vi "NagleDemo-MessageSender.vi"() -> ()   [LabVIEW 2014]
panel:
  in  "TCP_NODELAY":bool=TRUE caption="false: Nagle alg. ENABLED\ntrue: Nagle alg. DISABLED"
  in  "n iterations":i32=100
  in  "IP address of MessageReflector":string
  out "value":i32
  in  "remote port":u16=5678
  out "error out":errorcluster
  out "roundtrip time (ms)":u32(graph)
  # "This VI demonstrates the effect of having the TCP Nagle algorithm enabled or disabled on  a socket for a particular kind of query/response protocol.\n\nTo run this demo, first run its partner in crime, NagleDemo-MessageSender.vi, on another machine, then run this VI after filling in the IP address of the other machine. Between runs of this VI, toggle the TCP_NODELAY boolean to see the difference."
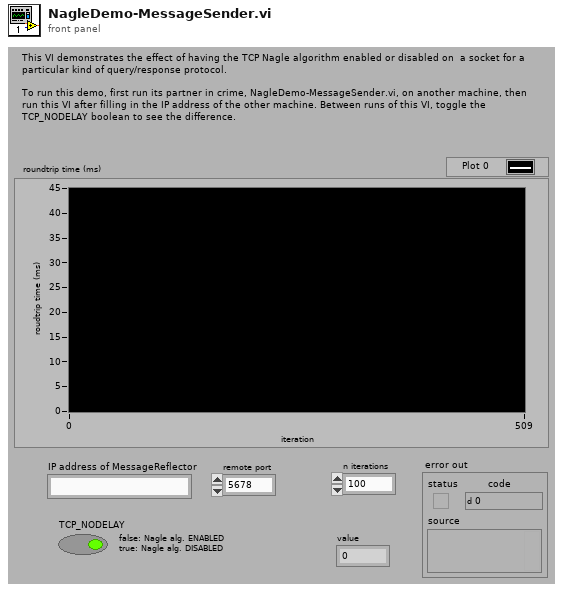
[diagram p1: front panel]
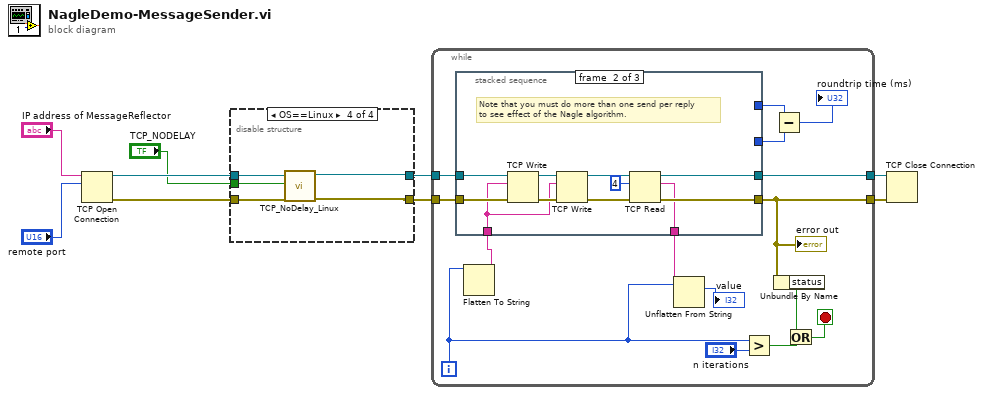
[diagram p0: block diagram]
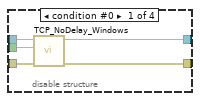
[diagram p2: hidden frame]
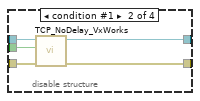
[diagram p3: hidden frame]
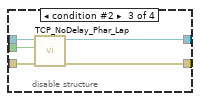
[diagram p4: hidden frame]
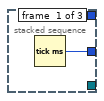
[diagram p5: hidden frame]
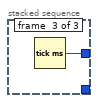
[diagram p6: hidden frame]
diagram:
  n1 = TCP Open Connection(address="IP address of MessageReflector", remote port or service name="remote port") -> (connection ID=w3:refnum<k5>, error out=w1:errorcluster)  [unwired: 3 in]
  n2 = disable-structure shown="OS==Linux" {
    disable-tunnel: [w14 w18 w23 w25] -> w5
    disable-tunnel: [w13 w17 w22 w26] -> w4
    disable-tunnel: w3 -> [w12 w16 w21 w28]
    disable-tunnel: "TCP_NODELAY" -> [w11 w15 w20 w27]
    disable-tunnel: w1 -> [w10 w19 w24 w29]
    frame condition #0 {
      n3 = call "TCP_NoDelay_Windows.vi"("error in (no error)"=w10, "TCP_NODELAY (true)"=w11, "connID"=w12) -> ("error out"=w14:errorcluster, "connID 2"=w13:refnum<k5>)  [unwired: 3 in]
    }
    frame condition #1 {
      n4 = call "TCP_NoDelay_VxWorks.vi"("error in (no error)"=w19, "TCP_NODELAY (true)"=w15, "connID"=w16) -> ("error out"=w18:errorcluster, "connID 2"=w17:refnum<k5>)  [unwired: 3 in]
    }
    frame condition #2 {
      n5 = call "TCP_NoDelay_Phar_Lap.vi"("error in (no error)"=w24, "TCP_NODELAY (true)"=w20, "connID"=w21) -> ("error out"=w23:errorcluster, "connID 2"=w22:refnum<k5>)  [unwired: 3 in]
    }
    frame condition #3 (active) {
      n6 = call "TCP_NoDelay_Linux.vi"("error in (no error)"=w29, "TCP_NODELAY (true)"=w27, "connID"=w28) -> ("error out"=w25:errorcluster, "connID 2"=w26:refnum<k5>)  [unwired: 3 in]
    }
  }
  n7 = while {
    tunnel: w4 -> [w44]
    tunnel: [w43] -> w9
    tunnel: [w39] -> w8
    tunnel: w5 -> [w42]
    i -> [w32]
    stop <- w35 stop-if-true
    n8 = Flatten To String(anything=w32) -> (data string=w34:string)  [unwired: 3 in, 2 out]
    n9 = stacked-sequence {
      tunnel: w44 -> [_ w56 _]
      tunnel: [_ w55 _] -> w43
      tunnel: w42 -> [_ w54 _]
      tunnel: [_ w52 _] -> w39
      tunnel: [w45 _ _] -> w40
      tunnel: [_ _ w57] -> w41
      tunnel: w34 -> [_ w46 _]
      tunnel: [_ w51 _] -> w33
      frame #0 {
        n10 = Tick Count (ms)() -> (millisecond timer value=w45:u32)
      }
      frame #1 {
        # "Note that you must do more than one send per reply\nto see effect of the Nagle algorithm."
        n11 = TCP Write(connection ID=w56, data in=w46, error in (no error)=w54) -> (connection ID out=w50:refnum<k5>, error out=w49:errorcluster)  [unwired: 1 in, 1 out]
        n12 = TCP Write(connection ID=w50, data in=w46, error in (no error)=w49) -> (connection ID out=w47:refnum<k5>, error out=w48:errorcluster)  [unwired: 1 in, 1 out]
        n13 = TCP Read(connection ID=w47, bytes to read=4, error in (no error)=w48) -> (connection ID out=w55:refnum<k5>, data out=w51:string, error out=w52:errorcluster)  [unwired: 2 in]
      }
      frame #2 {
        n14 = Tick Count (ms)() -> (millisecond timer value=w57:u32)
      }
    }
    "error out" <- w39
    n15 = Unflatten From String(type=w32, binary string=w33) -> (value=→"value":i32)  [unwired: 3 in, 2 out]
    n16 = Greater?(x=w32, y="n iterations") -> (0:w37:bool)
    n17 = Subtract(x=w41, y=w40) -> (x-y=→"roundtrip time (ms)":u32)
    n18 = Unbundle By Name(w39) -> ("status"=w36:bool)
    n19 = Or(x=w36, y=w37) -> (x .or. y?=w35:bool)
  }
  n20 = TCP Close Connection(connection ID=w9, error in (no error)=w8) -> ()  [unwired: 1 in, 2 out]
